vi "Check System Status.vi"(8 "error in (no error)":errorcluster, 11 "CIFCorePlugin in":refnum<class "CIFCorePlugin.lvclass">) -> (0 "error out":errorcluster, 3 "CIFCorePlugin out":refnum<class "CIFCorePlugin.lvclass">)   [LabVIEW 2021, in "CIFCorePlugin.lvclass"]
uses:
  CIFCorePlugin.lvclass
  CIFCorePlugin.lvclass/CIFCorePlugin.ctl
  CIFPluginManager/CIFPluginManager/gRPC/CIF_Manager_Client_Wrapper/CIFManagerClientWrapper.lvlib
  CIFUtilities/CIFClocks/CIFClocks.lvlib
  OOB/OOB_Rx/CIFCoreOOB_Rx.lvclass
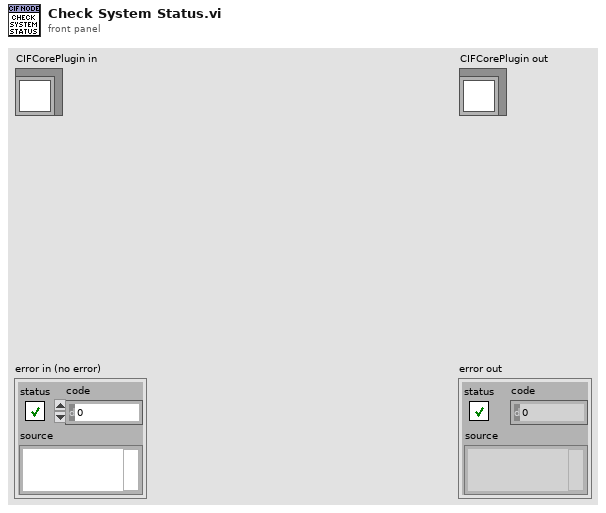
[diagram p1: front panel]
types:
  T1 = typedef "grpc-lvsupport-release.lvlib/grpcId.ctl" = u64
  T2 = typedef "CIFClocks.lvlib/Clock Conversion Map.ctl" = map{u8, cluster{"Last Reset":u64, "Offset Pair":T3, "Slope":dbl}}
  T3 = typedef "CIFClocks.lvlib/Timestamp Pair.ctl" = cluster{"System Time":i64, "External Time":i64}
  T4 = typedef "CIFCoreCommon.lvlib/Plugin Status.ctl" = cluster{"State":T5, "Timing Statistics (us)":T6, "FIFO Statistics (us)":T8, "error":T9, "Monitor Doubles":T10, "Monitor U64":T11, "Monitor I64":T12, "Cleanup":T7, "Create":i32, "Destroy":i32}
  T5 = typedef "CIFCoreCommon.lvlib/Plugin State.ctl" = enum32{"Null", "Creating", "Listening", "Running", "CleaningUp", "Destroying"}
  T6 = typedef "CIFCoreCommon.lvlib/Timing Statistics.ctl" = cluster{"Period":T7, "Wake Error":T7, "Execute":T7, "Housekeep":T7, "Idle":T7}
  T7 = typedef "CIFCoreCommon.lvlib/Timing Stats Base.ctl" = cluster{"Max":i32, "Min":i32}
  T8 = typedef "CIFCoreCommon.lvlib/FIFO Statistics.ctl" = cluster{"From T0":T7, "From Previous Plugin":T7, "Output Error":T7}
  T9 = typedef "CIFCoreCommon.lvlib/Simple Error.ctl" = cluster{"status":bool, "code":i32}
  T10 = typedef "CIFCoreCommon.lvlib/Monitor Doubles.ctl" = cluster{"1":dbl, "2":dbl, "3":dbl, "4":dbl}
  T11 = typedef "CIFCoreCommon.lvlib/Monitor U64.ctl" = cluster{"1":u64, "2":u64, "3":u64, "4":u64}
  T12 = typedef "CIFCoreCommon.lvlib/Monitor I64.ctl" = cluster{"1":i64, "2":i64, "3":i64, "4":i64}
  T13 = typedef "CIFClocks.lvlib/Clock Conversion.ctl" = cluster{"ClockID":u8, "Last Reset":u64, "Offset Pair":T3, "Slope":dbl, "Name":string}
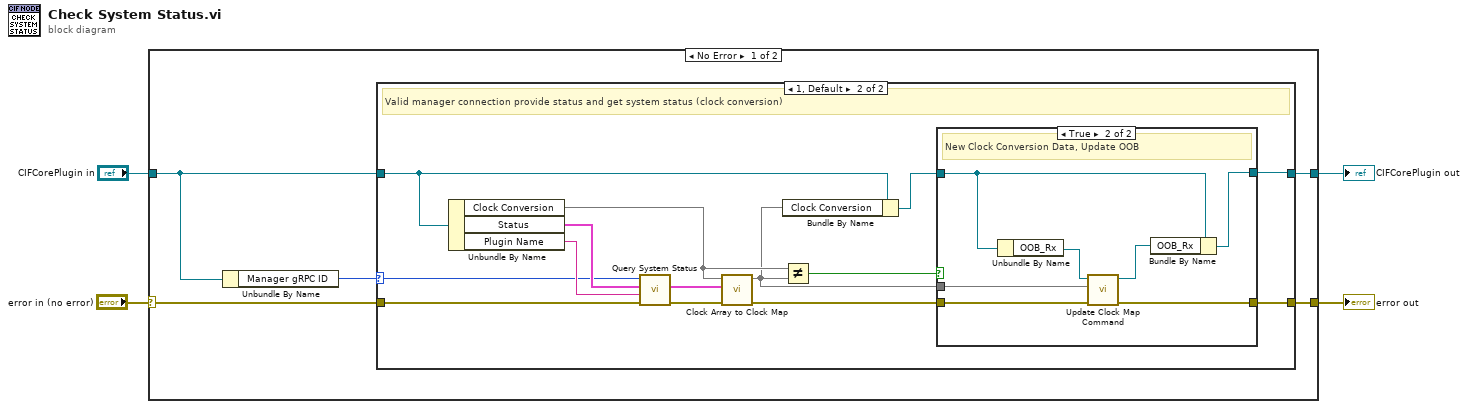
[diagram p0: block diagram]
diagram:
  n1 = case shown="No Error" "error in (no error)" {
    selector: "error in (no error)" -> [w5 w36]
    tunnel: [w9 w36] -> w3
    tunnel: [w8 w35] -> w1
    tunnel: "CIFCorePlugin in" -> [w7 w35]
    frame No Error {
      n2 = Unbundle By Name(w7) -> ("Manager gRPC ID"=w6:T1)
      n3 = case shown="1, Default" w6 {
        selector: w6 -> [_ w22]
        tunnel: [w11 w15] -> w9
        tunnel: [w10 w12] -> w8
        tunnel: w7 -> [w10 w21]
        tunnel: w5 -> [w11 w23]
        frame 0 {
          # "No connection to manager (development test mode)"
        }
        frame 1, Default {
          # "Valid manager connection provide status and get system status (clock conversion)"
          n4 = Unbundle By Name(w21) -> ("Clock Conversion"=w18:T2, "Status"=w25:T4, "Plugin Name"=w24:string)
          n5 = call "Query System Status.vi"("error in"=w23, "Plugin Name"=w24, "Status"=w25, "gRPC ID in"=w22) -> ("error out"=w20:errorcluster, "Clock Conversion Array"=w19:T13[])  [unwired: 5 in, 1 out]
          n6 = call "Clock Array to Clock Map.vi"("error in (no error)"=w20, "Clock Conversion Array"=w19, "Clock Convert Map in"=w18) -> ("error out"=w16:errorcluster, "Clock Convert Map out"=w13:T2)  [unwired: 7 in]
          n7 = Bundle By Name(cluster=w21, "Clock Conversion"=w13) -> (w14:refnum<class "CIFCorePlugin.lvclass">)
          n8 = Not Equal?(x=w18, y=w13) -> (x != y?=w17:bool)
          n9 = case shown="True" w17 {
            tunnel: w16 -> [w26 w34]
            tunnel: [w26 w33] -> w15
            tunnel: w14 -> [w27 w29]
            tunnel: w13 -> [_ w31]
            tunnel: [w27 w28] -> w12
            frame False {
            }
            frame True {
              # "New Clock Conversion Data, Update OOB"
              n10 = Unbundle By Name(w29) -> ("OOB_Rx"=w32:refnum<class "CIFCoreOOB_Rx.lvclass">)
              n11 = call "Update Clock Map Command.vi"("error in"=w34, "Clock Conversion"=w31, "CoreOOB_Rx in"=w32) -> ("error out"=w33:errorcluster, "CoreOOB_Rx out"=w30:refnum<class "CIFCoreOOB_Rx.lvclass">)  [unwired: 7 in]
              n12 = Bundle By Name(cluster=w29, "OOB_Rx"=w30) -> (w28:refnum<class "CIFCorePlugin.lvclass">)
            }
          }
        }
      }
    }
    frame Error {
    }
  }
  "error out" <- w3
  "CIFCorePlugin out" <- w1
